vi "Reset Pause Flag.vi"(8 "error in (no error)":errorcluster, 11 "Monkey in":refnum<class "Monkey.lvclass">) -> (0 "error out":errorcluster, 3 "Monkey out":refnum<class "Monkey.lvclass">)   [LabVIEW 2020, in "TALOS.lvlib" / "Monkey.lvlib" / "Monkey.lvclass"]
doc: "Negate the pause flag if the stopped flag wasn't raised. Show/hide indicator"
uses:
  Monkey.lvclass
  C:/LabVIEW Code/TALOS/talos/Father of all uServices/Father of all uServices/Father of all uServices.lvclass
  Monkey.lvclass/Monkey.ctl
  Father of all uServices/Father of all uServices/Father of all uServices.lvclass
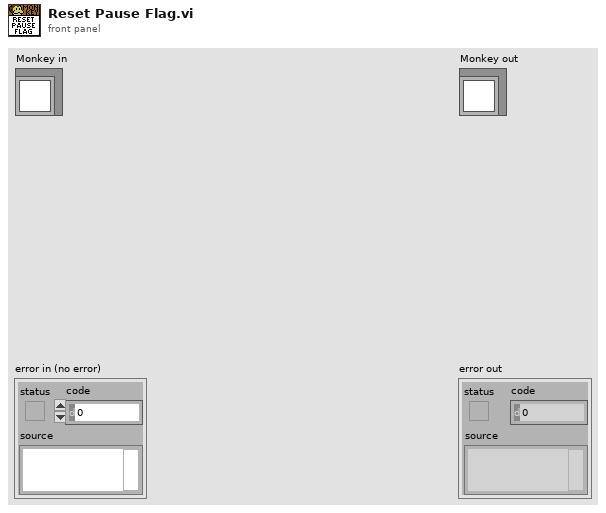
[diagram p1: front panel]
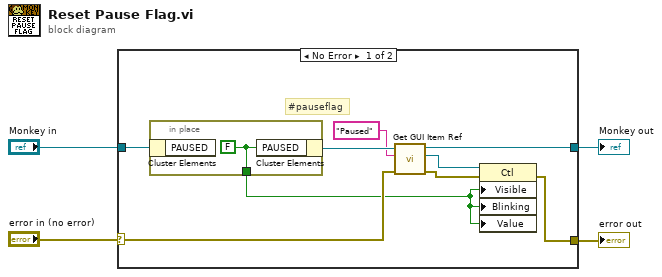
[diagram p0: block diagram]
diagram:
  n1 = case shown="No Error" "error in (no error)" {
    selector: "error in (no error)" -> [w10 w16]
    tunnel: [w12 w16] -> w3
    tunnel: [w13 w15] -> w1
    tunnel: "Monkey in" -> [w11 w15]
    frame No Error {
      # "#pauseflag"
      n2 = in-place {
        in-place-border: [w14] -> w5
        w14 = FALSE
        n3 = in-place-cluster #1(w11) -> ()  [unwired: 1 out]
        n4 = in-place-cluster #1("PAUSED"=w14) -> (w9:refnum<class "Monkey.lvclass">)
      }
      n5 = call "Get GUI Item Ref.vi"("error in (no error)"=w10, "FP Item Name"="Paused", "uService Template in"=w9) -> ("error out"=w6:errorcluster, "Ctl Refnum"=w7:refnum<vi>, "uService Template out"=w13:refnum<class "Monkey.lvclass">)  [unwired: 6 in]
      n6 = property class="Ctl"(reference=w7, error in=w6, "Visible"=w5, "Blinking"=w5, "Value"=w5) -> (error out=w12:errorcluster)  [unwired: 1 out]
    }
    frame Error {
    }
  }
  "error out" <- w3
  "Monkey out" <- w1
